vi "Read Driver Settings.vi"(8 "error in (no error)":errorcluster, 11 "Driver in":refnum<class "Driver.lvclass">) -> (0 "error out":errorcluster, 2 "Driver Settings":variant, 3 "Driver out":refnum<class "Driver.lvclass">)   [LabVIEW 2023, in "HAF.lvlib" / "Driver.lvclass"]
doc: "Returns all the Driver Settings held by this Driver. If the Driver Settings have not been set up, then it initialised the Variant.\n\nDriver Settings act like a Dictionary Data Type. The entries are stored as named attributes."
uses:
  Driver.lvclass
  <vilib>/Utility/Data Type/Type Definitions/Data Type.ctl
  Driver.lvclass/Driver.ctl
  DriverSetting/DriverSetting.lvclass
  <vilib>/Utility/Data Type/NI_Data Type.lvlib
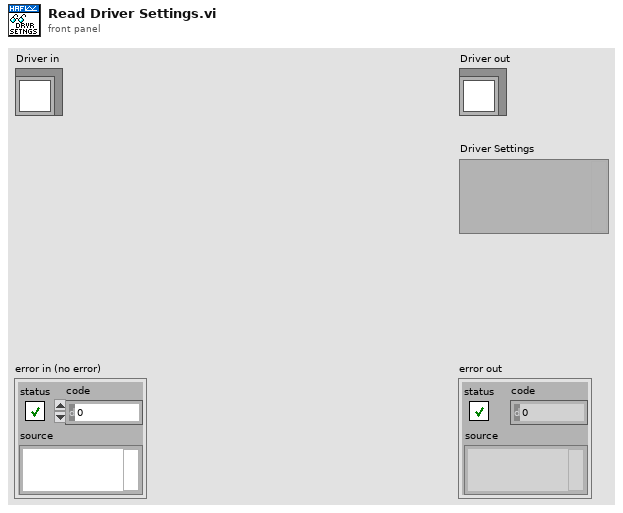
[diagram p1: front panel]
types:
  T1 = typedef "NI_Data Type.lvlib/Data Type.ctl" = enum8{"Invalid Type", "Void", "I8", "I16", "I32", "I64", "U8", "U16", "U32", "U64", "Single Float", "Double Float", "Extended Float", "Single Complex", "Double Complex", "Extended Complex", "Enum U8", "Enum U16", "Enum U32", "Enum U64", "Single Float With Unit", "Double Float With Unit", "Extended Float With Unit", "Single Complex with Unit", "Double Complex with Unit", "Extended Complex with Unit", "Boolean", "String", "Path", "Picture", "Tag", "Array", "Cluster", "Variant", "LV Variant", "Waveform", "Timestamp", "Digital Waveform", "Digital Data", "ExpressData", "Refnum", "External Data", "VI", "Poly VI", "LabVIEW Class Instance", "Fixed Point", "Set Collection", "Map Collection"}
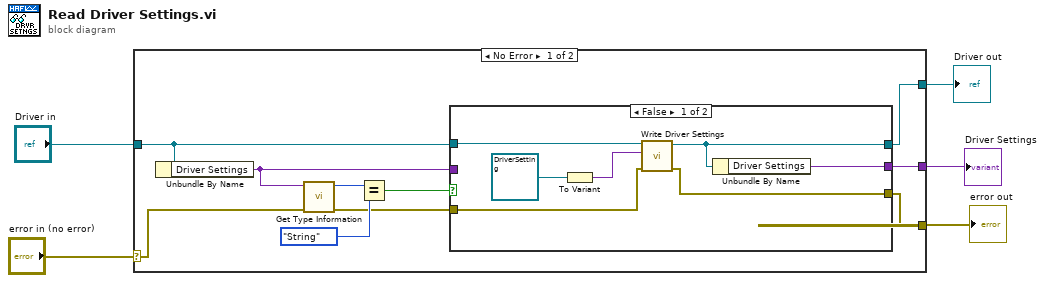
[diagram p0: block diagram]
diagram:
  n1 = case shown="No Error" "error in (no error)" {
    selector: "error in (no error)" -> [w15 w26]
    tunnel: [w6 w26] -> w4
    tunnel: [w8 w27] -> w2
    tunnel: "Driver in" -> [w9 w27]
    tunnel: [w7 _] -> w1
    frame No Error {
      n2 = Unbundle By Name(w9) -> ("Driver Settings"=w10:variant)
      n3 = call <vilib>:"Get Type Information.vi"("error in (no error)"=w15, "variant"=w10) -> ("error out"=w11:errorcluster, "type"=w14:T1)  [unwired: 5 in, 3 out]
      n4 = Equal?(x=w14, y=Data_Type."String") -> (x = y?=w12:bool)
      n5 = case shown="False" w12 {
        tunnel: w11 -> [w19 w23]
        tunnel: w10 -> [_ w24]
        tunnel: w9 -> [w21 w25]
        tunnel: [w16 w25] -> w8
        tunnel: [w17 w24] -> w7
        tunnel: [w18 w23] -> w6
        frame False {
          n6 = To Variant(anything=refnum<class "DriverSetting.lvclass"> refnum ("HAF:DriverSetting.lvclass")) -> (Variant=w20:variant)
          n7 = call-dynamic "Write Driver Settings.vi"("error in (no error)"=w19, "Driver Settings"=w20, "Driver in"=w21) -> ("error out"=w18:errorcluster, "Driver out"=w16:refnum<class "Driver.lvclass">)  [unwired: 7 in]
          n8 = Unbundle By Name(w16) -> ("Driver Settings"=w17:variant)
        }
        frame True {
        }
      }
    }
    frame Error {
    }
  }
  "error out" <- w4
  "Driver out" <- w2
  "Driver Settings" <- w1
